vi "UtilityLib.selectName.vi"(2 "names":string[](array[string]), 5 "error in (no error)":errorcluster) -> (16 "name":string, 17 "index":i32, 19 "error out":errorcluster)   [LabVIEW 2015, in "UtilityLib.lvlib"]
doc: "lets the user select a name from a string"
uses:
  UtilityLib.lvlib
panel:
  in  "Cancel":bool
  in  "OK Button":bool
  in  "Items":u16(ring)
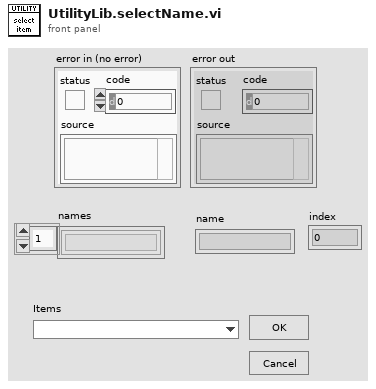
[diagram p1: front panel]
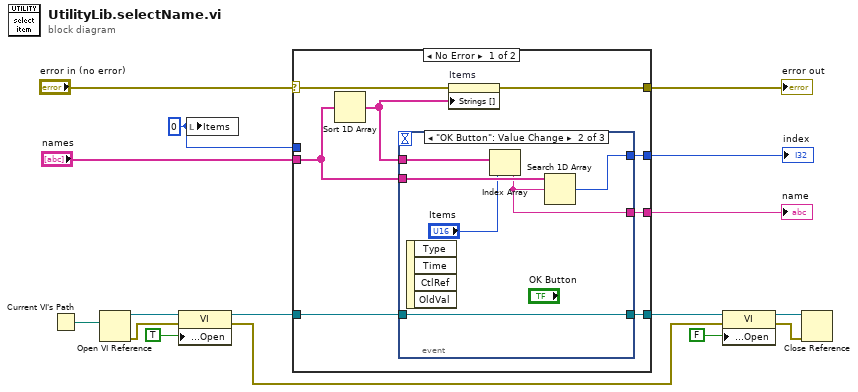
[diagram p0: block diagram]
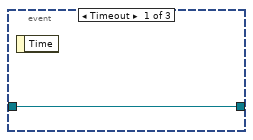
[diagram p2: hidden frame]
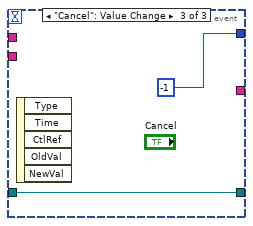
[diagram p3: hidden frame]
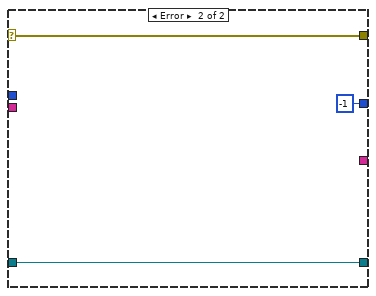
[diagram p4: hidden frame]
diagram:
  w1 = 0
  n1 = Current VI's Path() -> (path=w13:path)
  n2 = Open VI Reference(vi path=w13) -> (vi reference=w12:refnum<vi>, error out=w6:errorcluster)  [unwired: 5 in]
  n3 = property class="VI"(reference=w12, error in=w6, "Front Panel Window:Open"=TRUE) -> (reference out=w10:refnum<vi>, error out=w5:errorcluster)
  n4 = local write "Items"(w1) -> ()
  n5 = case shown="No Error" "error in (no error)" {
    selector: "error in (no error)" -> [w20 w36]
    tunnel: [w24 _] -> w16
    tunnel: "names" -> [w17 _]
    tunnel: [w23 w36] -> w14
    tunnel: w10 -> [w22 w35]
    tunnel: [w21 w35] -> w8
    tunnel: [w19 -1 ("Items")] -> w2
    tunnel: w1 -> [_ _]
    frame No Error {
      n6 = Sort 1D Array(array=w17) -> (sorted array=w18:string[])
      n7 = event shown="[1] \"OK Button\": Value Change" {
        selector: _ -> [_ _ _]
        dyn-events: _ -> [_ _ _]
        timeout: _ -> [_ _ _]
        tunnel: w18 -> [_ w31 _]
        tunnel: [_ w28 _] -> w24
        tunnel: [w25 w30 w33] -> w21
        tunnel: w22 -> [w25 w30 w33]
        tunnel: [_ w26 -1 ("Items")] -> w19
        tunnel: w17 -> [_ w29 _]
        event Timeout {
          n8 = event-data() -> ()  [unwired: 1 in, 1 out]
        }
        event "OK Button": Value Change {
          n9 = event-data() -> ()  [unwired: 1 in, 4 out]
          n10 = Index Array(array=w31, index="Items") -> (element=w28:string)
          n11 = Search 1D Array(1D array=w29, element=w28) -> (index of element=w26:i32)  [unwired: 1 in]
        }
        event "Cancel": Value Change {
          n12 = event-data() -> ()  [unwired: 1 in, 5 out]
        }
      }
      n13 = property on="Items" class="Ring (strict)"(error in=w20, "Strings []"=w18) -> (error out=w23:errorcluster)  [unwired: 1 in, 1 out]
    }
    frame Error {
    }
  }
  "error out" <- w14
  "name" <- w16
  "index" <- w2
  n14 = property class="VI"(reference=w8, error in=w5, "Front Panel Window:Open"=FALSE) -> (reference out=w7:refnum<vi>, error out=w4:errorcluster)
  n15 = Close Reference(reference=w7, error in (no error)=w4) -> ()  [unwired: 1 out]
